vi "Data.vi"(6 "Data Command":T1, 8 "error in":errorcluster) -> (0 "error out":errorcluster, 1 "Range error":bool, 2 "data rate (Hz)":dbl, 3 "Daq Name":string)   [LabVIEW 2015]
uses:
  Data cmd.ctl
  DAQ configuration/Sensor buffer command.ctl
  Stamp/stamp command.ctl
  <vilib>/DAQmx/read.llb/DAQmx Read (Analog 2D DBL NChan NSamp).vi
  <vilib>/Analysis/baseanly.llb/Mean (DBL).vi
  <vilib>/DAQmx/miscellaneous.llb/DAQmx Fill In Error Info.vi
  <vilib>/Analysis/NI_AALBase.lvlib
  <resource>/objmgr/daqmx.rc
panel:
  out "error after start":errorcluster
  out "error after stop":errorcluster
  out "AI voltage":dbl[](array[numeric])
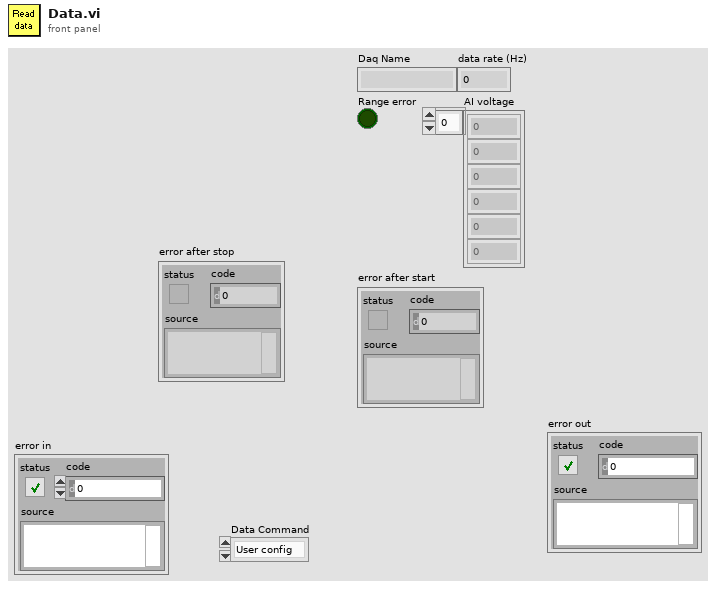
[diagram p1: front panel]
types:
  T1 = typedef "Data cmd.ctl" = enum16{"User config", "Ini config", "Read Data", "Close"}
  T2 = typedef "stamp command.ctl" = enum16{"Configure", "Write", "Off", "Close"}
  T3 = typedef "Sensor buffer command.ctl" = enum16{"read average", "read recent", "read all", "write", "set buffer size", "Read channel config", "Write channel config", "clear"}
  T4 = typedef "Channel config.ctl" = cluster{"Channel Indices":T5[], "AI Max voltage":dbl[], "Calibration matrix":T6}
  T5 = typedef "channel identifier.ctl" = u16
  T6 = typedef "calib array.ctl" = T7[]
  T7 = typedef "conversion.ctl" = cluster{"conversion matrix":sgl[][], "units":string, "name":string, "scale type":T8, "offset (volts)":dbl, "second channel":i8, "correspondence table":T9, "offset (physical units)":dbl, "pH scale":T10, "D.O.":T11, "Photometer data":T12}
  T8 = typedef "scale type.ctl" = enum16{"Volts", "Polynomial", "Correspondence Table", "pH", "Dissolved Oxygen", "Quadratic", "Photometer"}
  T9 = typedef "correspondence table.ctl" = cluster{"physical units":dbl, "volts":dbl}[]
  T10 = typedef "pH scale.ctl" = cluster{"Buffers":cluster{"Buffer":dbl, "Calibrated":bool, "V/T":dbl}[], "Temperature":dbl}
  T11 = typedef "DO scale.ctl" = cluster{"Temperature":dbl, "K":dbl, "barometric pressure":dbl}
  T12 = typedef "Photometer calibration data.ctl" = cluster{"Dark Voltage":dbl, "Blank Voltage":dbl, "Standards":cluster{"Concentration":dbl, "Voltage":dbl}[]}
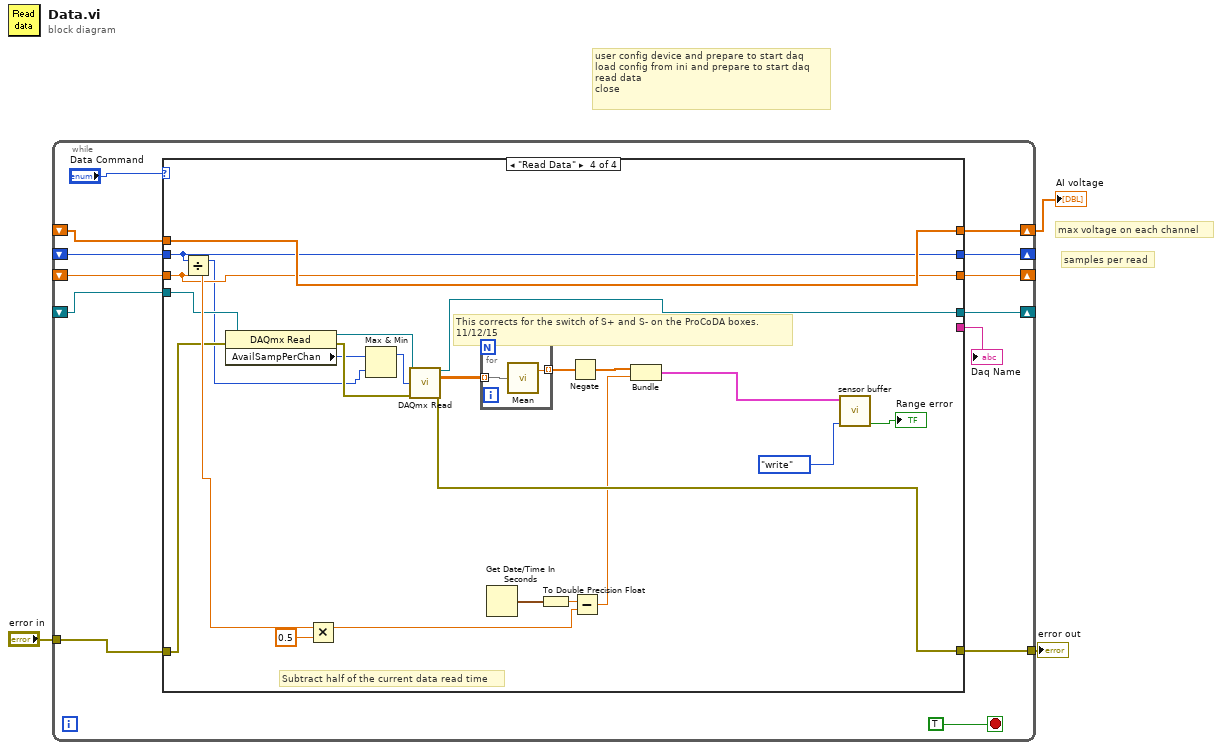
[diagram p0: block diagram]
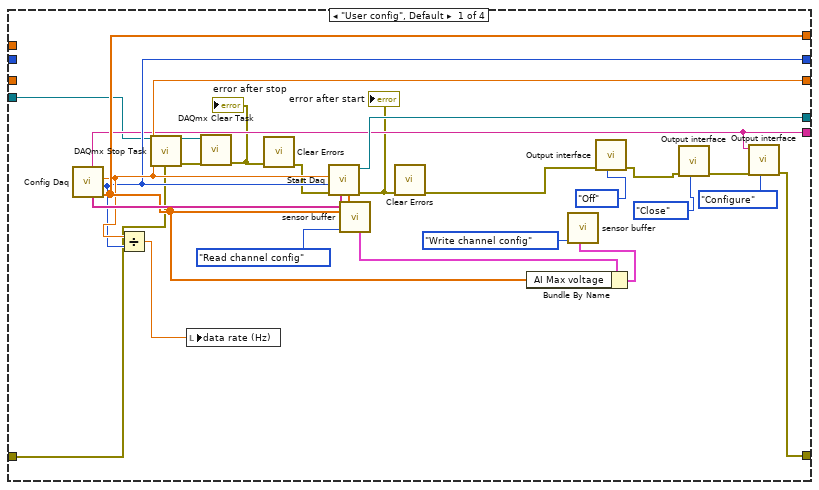
[diagram p2: hidden frame]
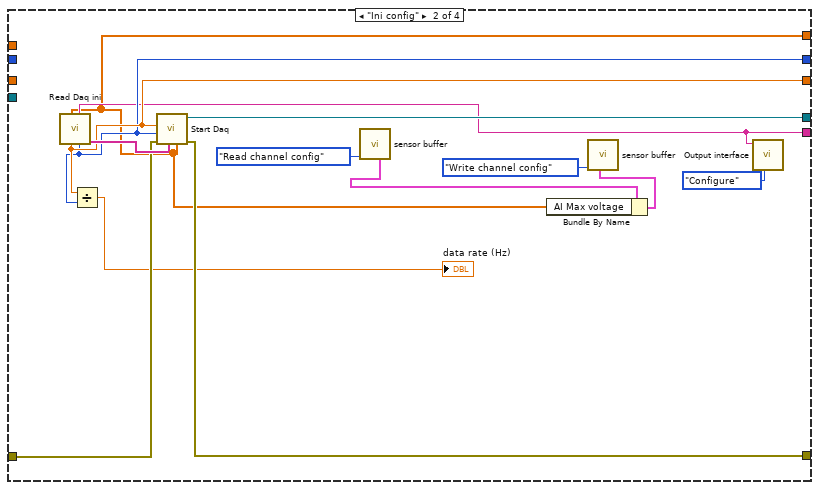
[diagram p3: hidden frame]
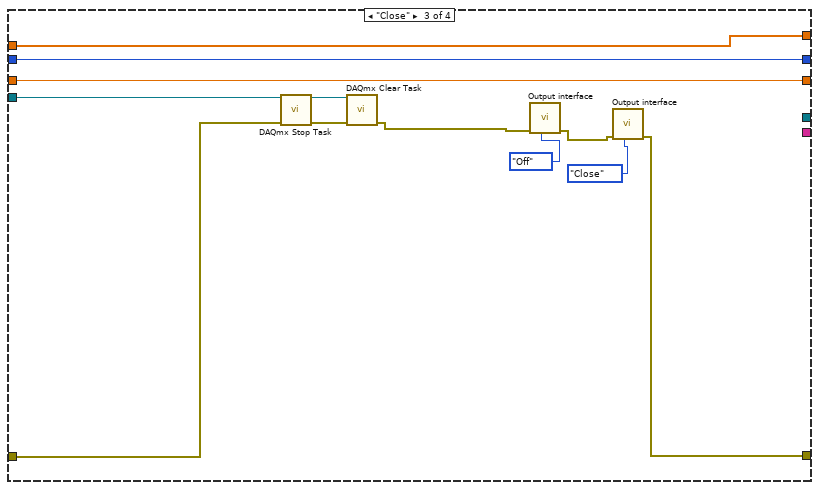
[diagram p4: hidden frame]
diagram:
  # "samples per read"
  # "max voltage on each channel"
  # "user config device and prepare to start daq\nload config from ini and prepare to start daq\nread data\nclose"
  n1 = while {
    tunnel: "error in" -> [w14]
    tunnel: [w13] -> w2
    shift-right: [w12] -> _
    shift-left: _ -> [w11]
    shift-right: [w10] -> w1
    shift-left: _ -> [w9]
    shift-right: [w8] -> _
    shift-left: _ -> [w7]
    shift-right: [w6] -> _
    shift-left: _ -> [w5]
    stop <- TRUE stop-if-true
    n2 = case shown="\"Read Data\"" "Data Command" {
      tunnel: w14 -> [w31 w54 w60 w72]
      tunnel: [w30 w53 w57 w80] -> w13
      tunnel: [w40 w52 _ w81] -> w12
      tunnel: w11 -> [w20 _ w62 w74]
      tunnel: [w35 w42 w67 w88] -> w10
      tunnel: w9 -> [_ _ w67 w88]
      tunnel: [w33 w46 w66 w69] -> w8
      tunnel: w7 -> [_ _ w66 w69]
      tunnel: [w34 w47 w65 w82] -> w6
      tunnel: w5 -> [_ _ w65 w82]
      tunnel: [w28 w43 _ _] -> w4
      frame "User config", Default {
        n3 = call "Config Daq.vi"() -> ("AI voltage"=w35:dbl[], "samples per read out"=w33:i32, "Data rate out (hz)"=w34:dbl, "AI Channels"=w41:string[], "Device Name"=w28:string)  [unwired: 6 in, 1 out]
        n4 = Divide(x=w34, y=w33) -> (x/y=w32:dbl)
        n5 = call <vilib>:"DAQmx Stop Task.vi"("task/channels in"=w20, "error in"=w31) -> ("task out"=w19:refnum<k21>, "error out"=w18:errorcluster)  [unwired: 12 in]
        n6 = local write "data rate (Hz)"(w32) -> ()
        n7 = call <vilib>:"DAQmx Clear Task.vi"("task in"=w19, "error in"=w18) -> ("error out"=w17:errorcluster)  [unwired: 13 in]
        "error after stop" <- w17
        n8 = call <vilib>:"Clear Errors.vi"("error in (no error)"=w17) -> ("error out"=w21:errorcluster)  [unwired: 5 in, 1 out]
        n9 = call "Start Daq.vi"("AI voltage"=w35, "AI Channels"=w41, "error in"=w21, "samples per read"=w33, "Data rate (hz)"=w34) -> ("error out"=w24:errorcluster, "task out"=w40:refnum<k21>)  [unwired: 5 in]
        "error after start" <- w24
        n10 = call "sensor buffer.vi"("command"=Sensor_buffer_command."Read channel config") -> ("Channel Config out"=w37:T4)  [unwired: 6 in, 4 out]
        n11 = call <vilib>:"Clear Errors.vi"("error in (no error)"=w24) -> ("error out"=w22:errorcluster)  [unwired: 5 in, 1 out]
        n12 = Bundle By Name(cluster=w37, "AI Max voltage"=w35) -> (w36:T4)
        n13 = call "sensor buffer.vi"("Channel Config"=w36, "command"=Sensor_buffer_command."Write channel config") -> ()  [unwired: 5 in, 5 out]
        n14 = call "Output interface.vi"("Stamp Command"=stamp_command."Off", "error in"=w22) -> ("error out"=w25:errorcluster)  [unwired: 8 in, 1 out]
        n15 = call "Output interface.vi"("Stamp Command"=stamp_command."Close", "error in"=w25) -> ("error out"=w27:errorcluster)  [unwired: 8 in, 1 out]
        n16 = call "Output interface.vi"("Stamp Command"=stamp_command."Configure", "error in"=w27, "DeviceName"=w28) -> ("error out"=w30:errorcluster)  [unwired: 7 in, 1 out]
      }
      frame "Ini config" {
        n17 = call "Read Daq ini.vi"() -> ("AI Channels"=w55:string[], "samples per read"=w46:i32, "DeviceName"=w43:string, "Data rate (hz)"=w47:dbl, "AI voltage"=w42:dbl[])  [unwired: 3 in, 4 out]
        n18 = Divide(x=w47, y=w46) -> (x/y=→"data rate (Hz)":dbl)
        n19 = call "Start Daq.vi"("AI voltage"=w42, "AI Channels"=w55, "error in"=w54, "samples per read"=w46, "Data rate (hz)"=w47) -> ("error out"=w53:errorcluster, "task out"=w52:refnum<k21>)  [unwired: 5 in]
        n20 = call "sensor buffer.vi"("command"=Sensor_buffer_command."Read channel config") -> ("Channel Config out"=w49:T4)  [unwired: 6 in, 4 out]
        n21 = Bundle By Name(cluster=w49, "AI Max voltage"=w42) -> (w48:T4)
        n22 = call "sensor buffer.vi"("Channel Config"=w48, "command"=Sensor_buffer_command."Write channel config") -> ()  [unwired: 5 in, 5 out]
        n23 = call "Output interface.vi"("Stamp Command"=stamp_command."Configure", "DeviceName"=w43) -> ()  [unwired: 8 in, 2 out]
      }
      frame "Close" {
        n24 = call <vilib>:"DAQmx Stop Task.vi"("task/channels in"=w62, "error in"=w60) -> ("task out"=w61:refnum<k21>, "error out"=w59:errorcluster)  [unwired: 12 in]
        n25 = call <vilib>:"DAQmx Clear Task.vi"("task in"=w61, "error in"=w59) -> ("error out"=w58:errorcluster)  [unwired: 13 in]
        n26 = call "Output interface.vi"("Stamp Command"=stamp_command."Off", "error in"=w58) -> ("error out"=w64:errorcluster)  [unwired: 8 in, 1 out]
        n27 = call "Output interface.vi"("Stamp Command"=stamp_command."Close", "error in"=w64) -> ("error out"=w57:errorcluster)  [unwired: 8 in, 1 out]
      }
      frame "Read Data" {
        # "This corrects for the switch of S+ and S- on the ProCoDA boxes.\n11/12/15"
        # "Subtract half of the current data read time"
        n28 = Divide(x=w69, y=w82) -> (x/y=w85:dbl)
        n29 = property class="DAQmx Read"(reference=w74, error in=w72) -> (reference out=w73:refnum<k21>, error out=w71:errorcluster, "AvailSampPerChan"=w70:u32)
        n30 = Multiply(x=w85, y=0.5) -> (x*y=w84:dbl)
        n31 = Max & Min(x=w70, y=w69) -> (max(x,y)=w68:u32)  [unwired: 1 out]
        n32 = call-poly <vilib>:"DAQmx Read.vi"("task/channels in"=w73, "number of samples per channel"=w68, "error in"=w71) -> ("task out"=w81:refnum<k21>, "data"=w87:dbl[][], "error out"=w80:errorcluster)  [unwired: 10 in]
        n33 = for {
          tunnel: w87 -> [w92] mode=indexing
          tunnel: [w91] -> w79 mode=indexing
          n34 = call-poly <vilib>:"Mean.vi"("X"=w92) -> ("mean"=w91:dbl)  [unwired: 1 out]
        }
        n35 = Get Date/Time In Seconds() -> (seconds since 1Jan1904=w90:timestamp)
        n36 = To Double Precision Float(number=w90) -> (double precision float=w86:dbl)
        n37 = Negate(x=w79) -> (-x=w75:dbl[])
        n38 = Subtract(x=w86, y=w84) -> (x-y=w78:dbl)
        n39 = Bundle(w75, w78) -> (w77:cluster{dbl[], dbl})  [unwired: 1 in]
        n40 = call "sensor buffer.vi"("command"=Sensor_buffer_command."write", "raw Data"=w77) -> ("Range error"=→"Range error":bool)  [unwired: 5 in, 4 out]
      }
    }
    "Daq Name" <- w4
  }
  "error out" <- w2
  "AI voltage" <- w1
